vi "Read Data Config.vi"(8 "error in (no error)":errorcluster, 11 "MassSpectrumExtractor in":refnum<class "MassSpectrumExtractor.lvclass">) -> (0 "error out":errorcluster, 2 "Extracted Data Info":cluster{"Name":string, "Config":variant}[](array[cluster]), 3 "MassSpectrumExtractor out":refnum<class "MassSpectrumExtractor.lvclass">)   [LabVIEW 2014, in "MassSpectrumExtractor.lvclass"]
uses:
  MassSpectrumExtractor.lvclass
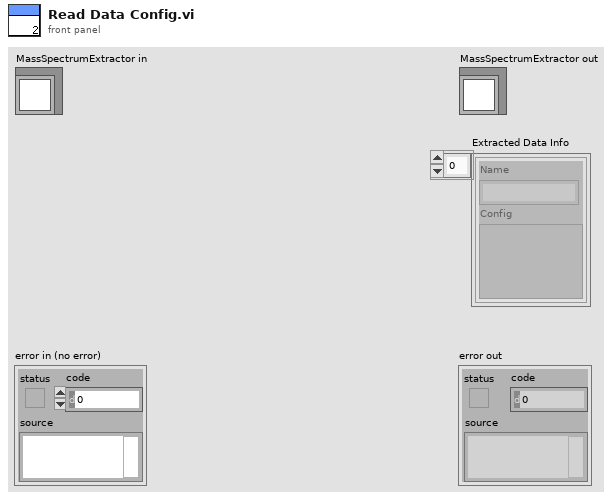
[diagram p1: front panel]
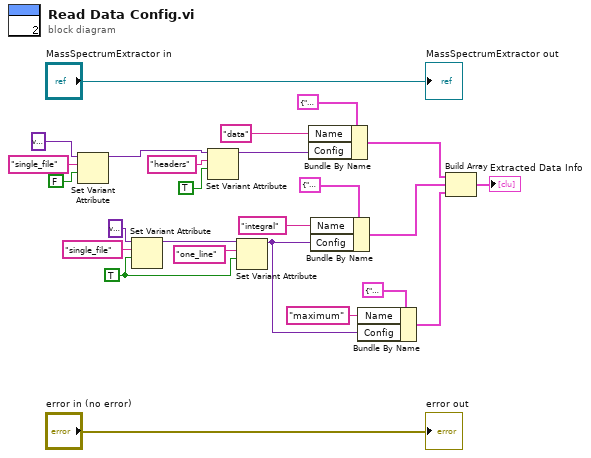
[diagram p0: block diagram]
diagram:
  w9 = TRUE ("Save to single file")
  n1 = Set Variant Attribute(Variant=variant ("variant"), name="single_file", value=FALSE ("Save to single file")) -> (Variant out=w8:variant)  [unwired: 1 in, 2 out]
  n2 = Set Variant Attribute(Variant=variant ("variant"), name="single_file", value=w9) -> (Variant out=w18:variant)  [unwired: 1 in, 2 out]
  n3 = Set Variant Attribute(Variant=w8, name="headers", value=TRUE ("Save to single file")) -> (Variant out=w7:variant)  [unwired: 1 in, 2 out]
  n4 = Set Variant Attribute(Variant=w18, name="one_line", value=w9) -> (Variant out=w3:variant)  [unwired: 1 in, 2 out]
  n5 = Bundle By Name(cluster=cluster{"Name":string, "Config":variant} {"Name"="", "Config"=variant} ("Cluster"), "Name"="data", "Config"=w7) -> (w12:cluster{"Name":string, "Config":variant})
  n6 = Bundle By Name(cluster=cluster{"Name":string, "Config":variant} {"Name"="", "Config"=variant} ("Cluster"), "Name"="integral", "Config"=w3) -> (w11:cluster{"Name":string, "Config":variant})
  n7 = Bundle By Name(cluster=cluster{"Name":string, "Config":variant} {"Name"="", "Config"=variant} ("Cluster"), "Name"="maximum", "Config"=w3) -> (w1:cluster{"Name":string, "Config":variant})
  n8 = Build Array(w12, w11, w1) -> (→"Extracted Data Info":cluster{"Name":string, "Config":variant}[])
  "error out" <- "error in (no error)"
  "MassSpectrumExtractor out" <- "MassSpectrumExtractor in"
